vi "CRC16_CCITT.vi"(6 "CRC_Mode":enum16{"CRC16", "CRC-16 (Modbus)"}(ring), 9 "sDt":string, 10 "iDt":u8[](array[numeric])) -> (1 "CRC":string, 2 "CRC16_LH":string, 4 "crc":u16 format="%x")   [LabVIEW 2015]
panel:
  out "crc_3":u16 format="%x"
  out "crc_1":u16 format="%x"
  out "CRCHi":u8 format="%.0x"
  out "CRCLo":u8 format="%.0x"
  out "crc_0":u16 format="%x"
  out "crc_0":u16 format="%x"
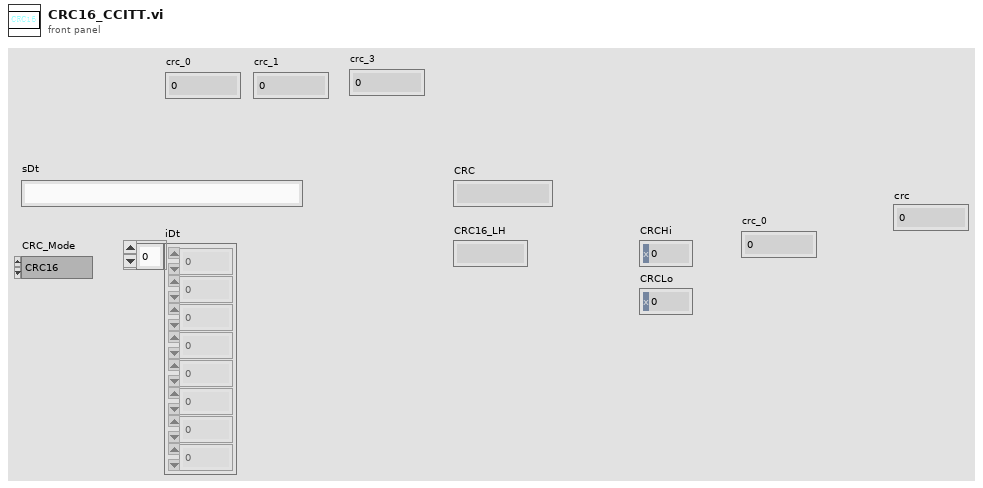
[diagram p1: front panel]
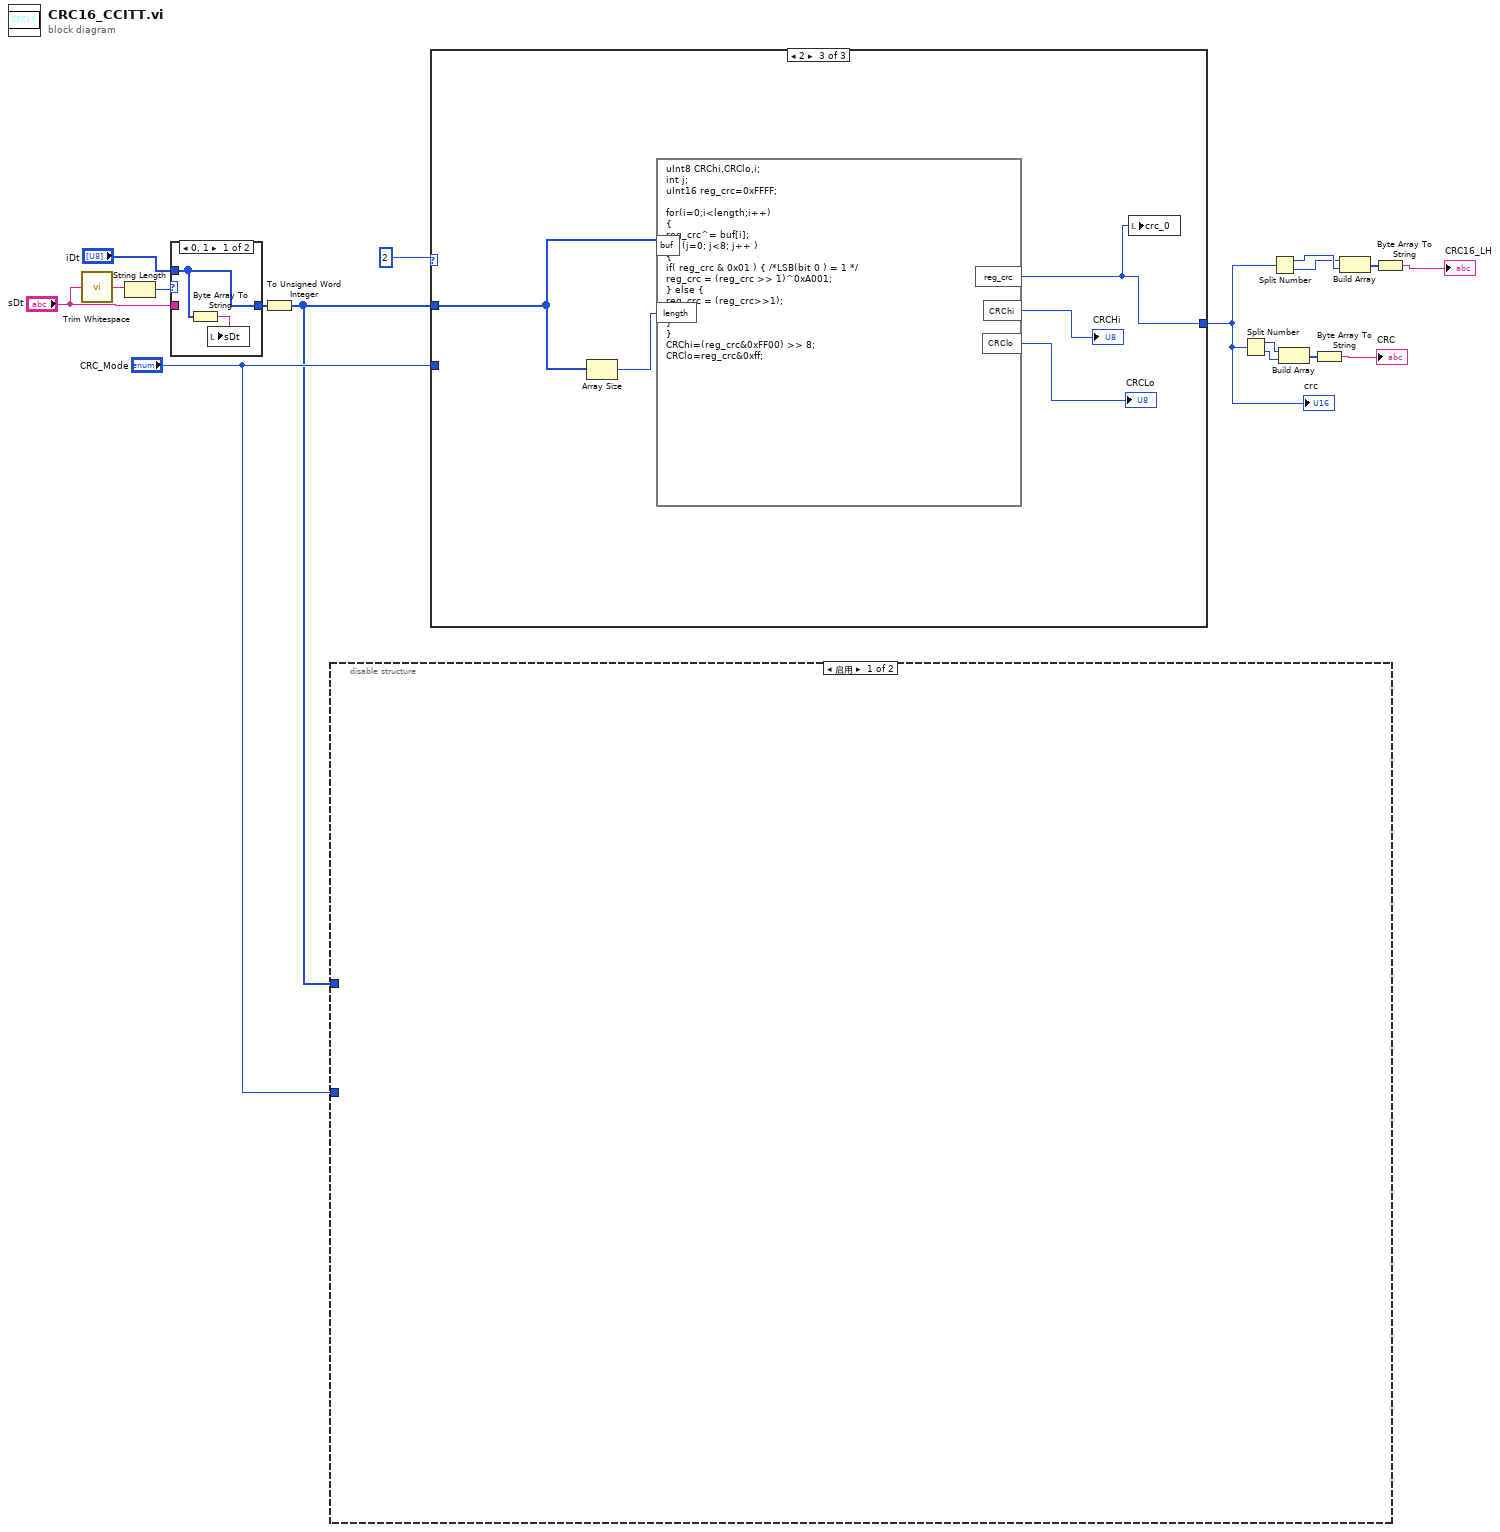
[diagram p0: block diagram]
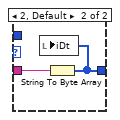
[diagram p2: hidden frame]
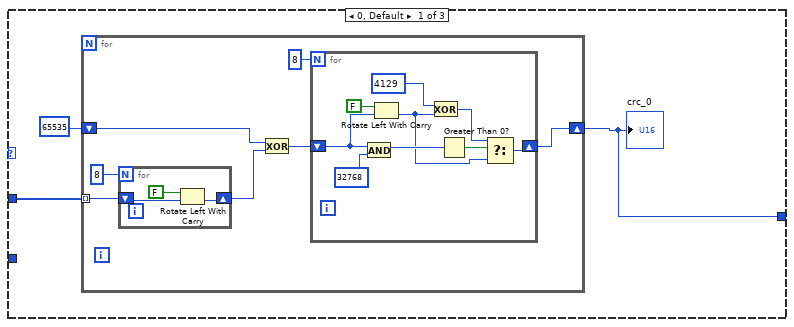
[diagram p3: hidden frame]
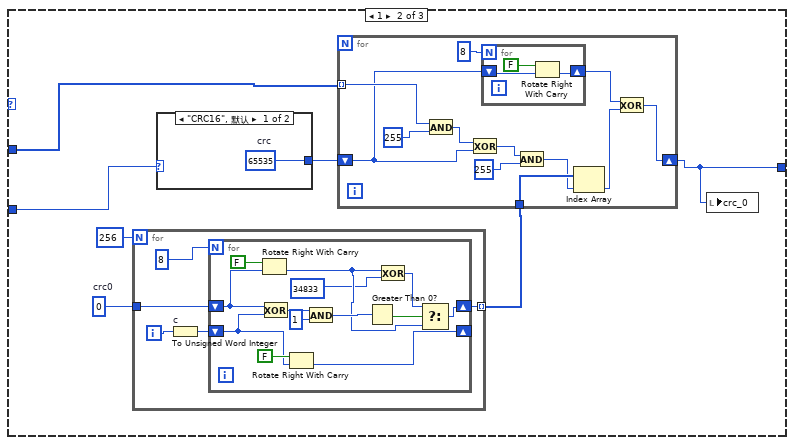
[diagram p4: hidden frame]
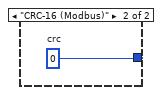
[diagram p5: hidden frame]
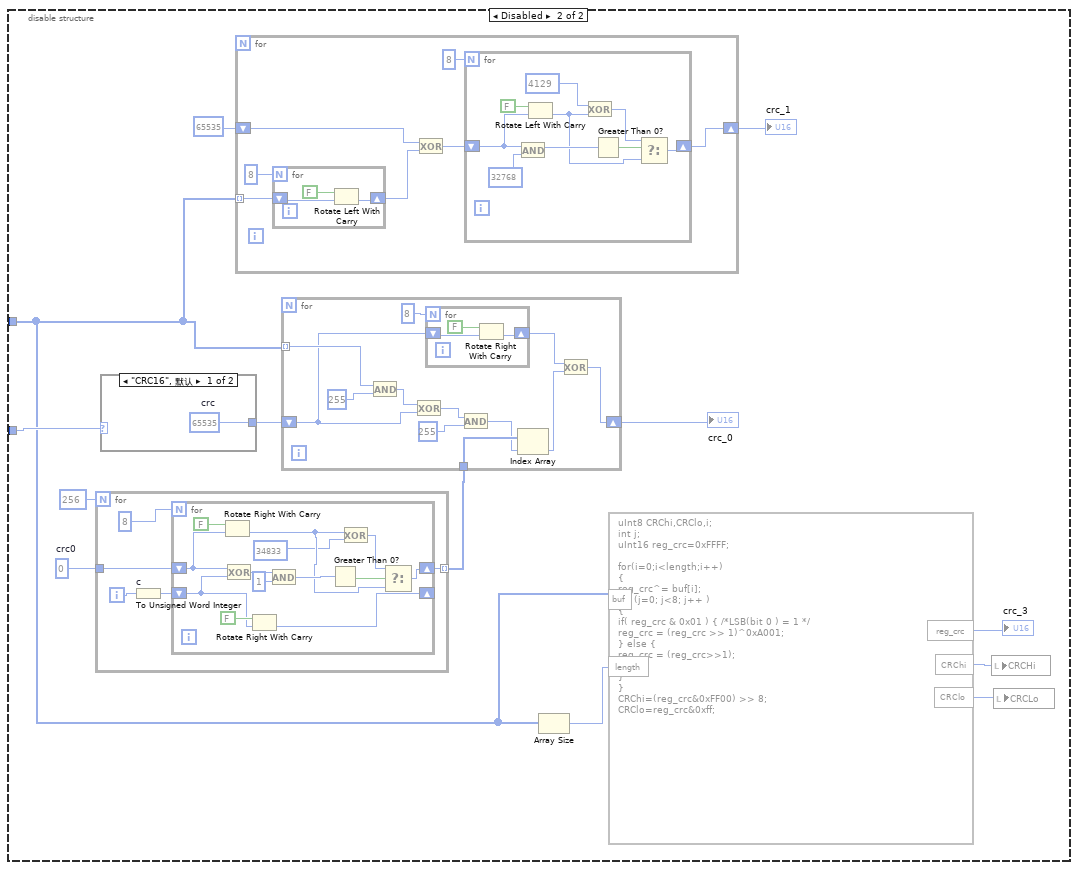
[diagram p6: hidden frame]
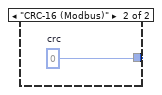
[diagram p7: hidden frame]
diagram:
  n1 = call <vilib>:"Trim Whitespace.vi"("string"="sDt") -> ("trimmed string"=w4:string)  [unwired: 1 in]
  n2 = String Length(string=w4) -> (length=w3:i32)
  n3 = case shown="0, 1" w3 {
    tunnel: [w19 w20] -> w17
    tunnel: "sDt" -> [_ w21]
    tunnel: "iDt" -> [w19 _]
    frame 0, 1 {
      n4 = Byte Array To String(unsigned byte array=w19) -> (string=w18:string)
      n5 = local write "sDt"(w18) -> ()
    }
    frame 2, Default {
      n6 = String To Byte Array(string=w21) -> (unsigned byte array=w20:u8[])
      n7 = local write "iDt"(w20) -> ()
    }
  }
  n8 = To Unsigned Word Integer(number=w17) -> (unsigned 16bit integer=w1:u16[])
  n9 = disable-structure shown="启用" {
    disable-tunnel: "CRC_Mode" -> [_ w32]
    disable-tunnel: w1 -> [_ w25]
    frame Enabled {
    }
    frame Disabled {
      w30 = u16 0  # crc0
      n10 = for {
        N: 256 -> [_]
        tunnel: w30 -> [w57]
        tunnel: [w54] -> w29 mode=indexing
        i -> [w56]
        n11 = To Unsigned Word Integer "c"(number=w56) -> (unsigned 16bit integer=w55:u16)
        n12 = for {
          N: 8 -> [_]
          shift-right: [w60] -> w54
          shift-left: w57 -> [w67]
          shift-right: [w62] -> _
          shift-left: w55 -> [w61]
          n13 = Rotate Right With Carry(2:w67, 3:FALSE ("进位")) -> (0:w65:u16)  [unwired: 1 out]
          n14 = Exclusive Or(1:w61, 2:w67) -> (0:w71:u16)
          n15 = Rotate Right With Carry(2:w61, 3:FALSE ("进位")) -> (0:w62:u16)  [unwired: 1 out]
          n16 = And(x=w71, y=u16 1) -> (x .and. y?=w69:u16)
          n17 = Greater Than 0?(x=w69) -> (x > 0?=w66:bool)
          n18 = Exclusive Or(1:u16 34833, 2:w65) -> (0:w64:u16)
          n19 = Select(t=w64, s=w66, f=w65) -> (s? t:f=w60:u16)
        }
      }
      n20 = case shown="\"CRC16\", 默认" w32 {
        tunnel: [w72 w73] -> w33
        frame "CRC16", Default {
          w72 = u16 65535  # crc
        }
        frame "CRC-16 (Modbus)" {
          w73 = u16 0  # crc
        }
      }
      n21 = for {
        tunnel: w25 -> [w40] mode=indexing
        shift-right: [w35] -> w27
        shift-left: u16 65535 -> [w38]
        n22 = for {
          N: 8 -> [_]
          shift-right: [w51] -> w39
          shift-left: w40 -> [w52]
          n23 = Rotate Left With Carry(2:w52, 3:FALSE ("进位")) -> (0:w51:u16)  [unwired: 1 out]
        }
        n24 = Exclusive Or(1:w39, 2:w38) -> (0:w37:u16)
        n25 = for {
          N: 8 -> [_]
          shift-right: [w42] -> w35
          shift-left: w37 -> [w44]
          n26 = And(x=w44, y=u16 32768 ("crc")) -> (x .and. y?=w49:u16)
          n27 = Rotate Left With Carry(2:w44, 3:FALSE ("进位")) -> (0:w43:u16)  [unwired: 1 out]
          n28 = Exclusive Or(1:w43, 2:u16 4129) -> (0:w45:u16)
          n29 = Greater Than 0?(x=w49) -> (x > 0?=w48:bool)
          n30 = Select(t=w45, s=w48, f=w43) -> (s? t:f=w42:u16)
        }
      }
      "crc_1" <- w27
      n31 = for {
        tunnel: w25 -> [w84] mode=indexing
        shift-right: [w74] -> w34
        shift-left: w33 -> [w81]
        tunnel: w29 -> [w80]
        n32 = And(x=w84, y=u16 255 ("crc")) -> (x .and. y?=w83:u16)
        n33 = Exclusive Or(1:w81, 2:w83) -> (0:w78:u16)
        n34 = for {
          N: 8 -> [_]
          shift-right: [w86] -> w76
          shift-left: w81 -> [w87]
          n35 = Rotate Right With Carry(2:w87, 3:FALSE ("进位")) -> (0:w86:u16)  [unwired: 1 out]
        }
        n36 = And(x=w78, y=u16 255 ("crc")) -> (x .and. y?=w77:u16)
        n37 = Index Array(array=w80, index=w77) -> (element=w75:u16)
        n38 = Exclusive Or(1:w75, 2:w76) -> (0:w74:u16)
      }
      "crc_0" <- w34
      n39 = Array Size(array=w25) -> (size(s)=w26:i32)
      n40 = formula code="uInt8 CRChi,CRClo,i;\nint j; \nuInt16 reg_crc=0xFFFF; \n \nfor(i=0;i<length;i++) \n{ \nreg_crc^= buf[i]; \nfor (j=0; j<8; j++ ) \n{ \nif( reg_crc & 0x01 ) { /*LSB(bit 0 ) = 1 */ \nreg_crc = (reg_crc >> 1)^0xA001; \n} else { \nreg_crc = (reg_crc>>1); \n} \n} \n} \nCRChi=(reg_crc&0xFF00) >> 8;\nCRClo=reg_crc&0xff;"("buf"=w25, "length"=w26) -> ("reg_crc"=→"crc_3":u16, "CRChi"=w23:u8, "CRClo"=w22:u8)
      n41 = local write "CRCHi"(w23) -> ()
      n42 = local write "CRCLo"(w22) -> ()
    }
  }
  n43 = case shown="2" i16 2 {
    tunnel: w1 -> [w90 w112 w154]
    tunnel: [w89 w111 w153] -> w8
    tunnel: "CRC_Mode" -> [_ w113 _]
    frame 0, Default {
      n44 = for {
        tunnel: w90 -> [w97] mode=indexing
        shift-right: [w92] -> w89
        shift-left: u16 65535 -> [w95]
        n45 = for {
          N: 8 -> [_]
          shift-right: [w108] -> w96
          shift-left: w97 -> [w109]
          n46 = Rotate Left With Carry(2:w109, 3:FALSE ("进位")) -> (0:w108:u16)  [unwired: 1 out]
        }
        n47 = Exclusive Or(1:w96, 2:w95) -> (0:w94:u16)
        n48 = for {
          N: 8 -> [_]
          shift-right: [w99] -> w92
          shift-left: w94 -> [w101]
          n49 = And(x=w101, y=u16 32768 ("crc")) -> (x .and. y?=w106:u16)
          n50 = Rotate Left With Carry(2:w101, 3:FALSE ("进位")) -> (0:w100:u16)  [unwired: 1 out]
          n51 = Exclusive Or(1:w100, 2:u16 4129) -> (0:w102:u16)
          n52 = Greater Than 0?(x=w106) -> (x > 0?=w105:bool)
          n53 = Select(t=w102, s=w105, f=w100) -> (s? t:f=w99:u16)
        }
      }
      "crc_0" <- w89
    }
    frame 1 {
      w115 = u16 0  # crc0
      n54 = for {
        N: 256 -> [_]
        tunnel: w115 -> [w121]
        tunnel: [w118] -> w114 mode=indexing
        i -> [w120]
        n55 = To Unsigned Word Integer "c"(number=w120) -> (unsigned 16bit integer=w119:u16)
        n56 = for {
          N: 8 -> [_]
          shift-right: [w124] -> w118
          shift-left: w121 -> [w131]
          shift-right: [w126] -> _
          shift-left: w119 -> [w125]
          n57 = Rotate Right With Carry(2:w131, 3:FALSE ("进位")) -> (0:w129:u16)  [unwired: 1 out]
          n58 = Exclusive Or(1:w125, 2:w131) -> (0:w135:u16)
          n59 = Rotate Right With Carry(2:w125, 3:FALSE ("进位")) -> (0:w126:u16)  [unwired: 1 out]
          n60 = And(x=w135, y=u16 1) -> (x .and. y?=w133:u16)
          n61 = Greater Than 0?(x=w133) -> (x > 0?=w130:bool)
          n62 = Exclusive Or(1:u16 34833, 2:w129) -> (0:w128:u16)
          n63 = Select(t=w128, s=w130, f=w129) -> (s? t:f=w124:u16)
        }
      }
      n64 = case shown="\"CRC16\", 默认" w113 {
        tunnel: [w136 w137] -> w117
        frame "CRC16", Default {
          w136 = u16 65535  # crc
        }
        frame "CRC-16 (Modbus)" {
          w137 = u16 0  # crc
        }
      }
      n65 = for {
        tunnel: w112 -> [w148] mode=indexing
        shift-right: [w138] -> w111
        shift-left: w117 -> [w145]
        tunnel: w114 -> [w144]
        n66 = And(x=w148, y=u16 255 ("crc")) -> (x .and. y?=w147:u16)
        n67 = Exclusive Or(1:w145, 2:w147) -> (0:w142:u16)
        n68 = for {
          N: 8 -> [_]
          shift-right: [w150] -> w140
          shift-left: w145 -> [w151]
          n69 = Rotate Right With Carry(2:w151, 3:FALSE ("进位")) -> (0:w150:u16)  [unwired: 1 out]
        }
        n70 = And(x=w142, y=u16 255 ("crc")) -> (x .and. y?=w141:u16)
        n71 = Index Array(array=w144, index=w141) -> (element=w139:u16)
        n72 = Exclusive Or(1:w139, 2:w140) -> (0:w138:u16)
      }
      n73 = local write "crc_0"(w111) -> ()
    }
    frame 2 {
      n74 = Array Size(array=w154) -> (size(s)=w157:i32)
      n75 = formula code="uInt8 CRChi,CRClo,i;\nint j; \nuInt16 reg_crc=0xFFFF; \n \nfor(i=0;i<length;i++) \n{ \nreg_crc^= buf[i]; \nfor (j=0; j<8; j++ ) \n{ \nif( reg_crc & 0x01 ) { /*LSB(bit 0 ) = 1 */ \nreg_crc = (reg_crc >> 1)^0xA001; \n} else { \nreg_crc = (reg_crc>>1); \n} \n} \n} \nCRChi=(reg_crc&0xFF00) >> 8;\nCRClo=reg_crc&0xff;"("buf"=w154, "length"=w157) -> ("reg_crc"=w153:u16, "CRChi"=→"CRCHi":u8, "CRClo"=→"CRCLo":u8)
      n76 = local write "crc_0"(w153) -> ()
    }
  }
  "crc" <- w8
  n77 = Split Number(x=w8) -> (hi(x)=w15:u8, lo(x)=w14:u8)
  n78 = Split Number(x=w8) -> (hi(x)=w13:u8, lo(x)=w12:u8)
  n79 = Build Array(w15, w14) -> (w16:u8[])
  n80 = Byte Array To String(unsigned byte array=w16) -> (string=→"CRC":string)
  n81 = Build Array(w12, w13) -> (w11:u8[])
  n82 = Byte Array To String(unsigned byte array=w11) -> (string=→"CRC16_LH":string)
